vi "Write Destination.vi"(8 "error in (no error)":errorcluster, 10 "Actor Framework:Message Enqueuer":refnum<class "Message Enqueuer.lvclass">, 11 "Analyze Actor in":refnum<class "Analyze Actor.lvclass">) -> (0 "error out":errorcluster, 3 "Analyze Actor out":refnum<class "Analyze Actor.lvclass">)   [LabVIEW 2014, in "Analyze Actor.lvlib" / "Analyze Actor.lvclass"]
uses:
  Analyze Actor.lvclass
  <vilib>/ActorFramework/Message Enqueuer/Message Enqueuer.lvclass
  Analyze Actor.lvclass/Analyze Actor.ctl
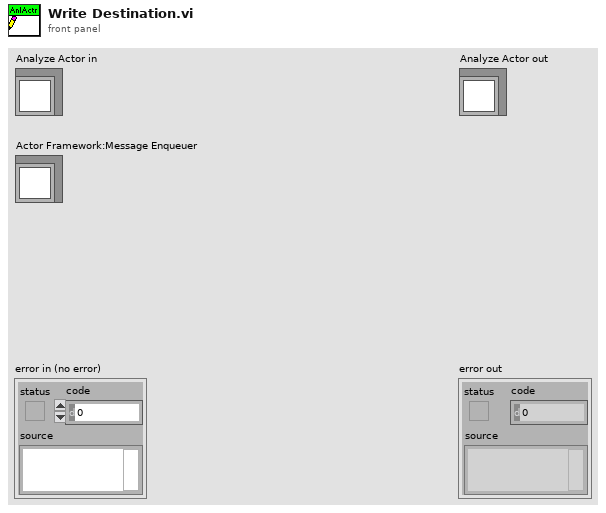
[diagram p1: front panel]
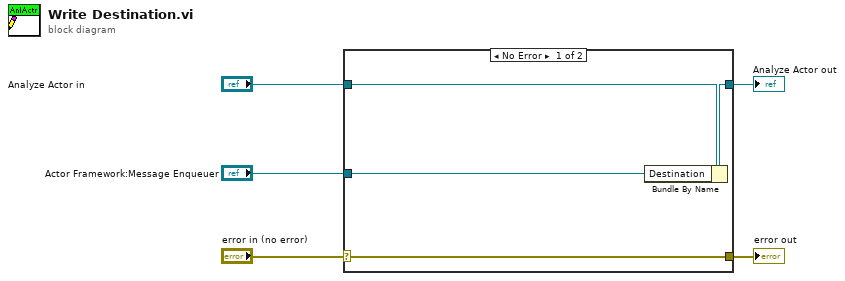
[diagram p0: block diagram]
diagram:
  n1 = case shown="No Error" "error in (no error)" {
    selector: "error in (no error)" -> [w9 w10]
    tunnel: [w9 w10] -> w4
    tunnel: [w7 w11] -> w2
    tunnel: "Analyze Actor in" -> [w8 w11]
    tunnel: "Actor Framework:Message Enqueuer" -> [w6 _]
    frame No Error {
      n2 = Bundle By Name(cluster=w8, "Destination"=w6) -> (w7:refnum<class "Analyze Actor.lvclass">)
    }
    frame Error {
    }
  }
  "error out" <- w4
  "Analyze Actor out" <- w2
